vi "WPI_Camera FPS Met.vi"(5 "robot fps":i32 min=0 step=1, 9 "dashboard fps":i32 min=0 step=1) -> (6 "robot fps met?":bool, 10 "dashboard fps met?":bool)   [LabVIEW 2017]
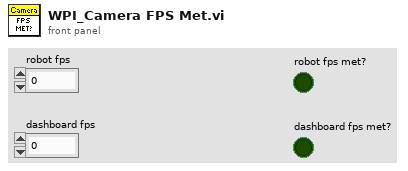
[diagram p1: front panel]
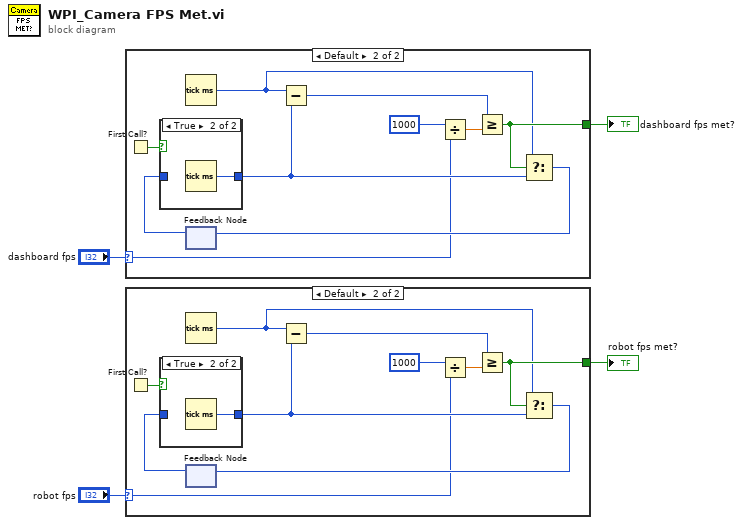
[diagram p0: block diagram]
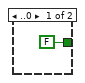
[diagram p2: hidden frame]
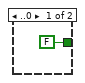
[diagram p4: hidden frame]
diagram:
  n1 = case shown="Default" "dashboard fps" {
    selector: "dashboard fps" -> [_ w6]
    tunnel: [FALSE w10] -> w4
    frame ..0 {
    }
    frame Default {
      n2 = First Call?() -> (First Call?: T/F=w15:bool)
      n3 = Tick Count (ms)() -> (millisecond timer value=w9:u32)
      n4 = feedback #1() -> (w14:u32)  [unwired: 1 in]
      n5 = case shown="True" w15 {
        tunnel: [w16 w17] -> w7
        tunnel: w14 -> [w16 _]
        frame False {
        }
        frame True {
          n6 = Tick Count (ms)() -> (millisecond timer value=w17:u32)
        }
      }
      n7 = Subtract(x=w9, y=w7) -> (x-y=w11:u32)
      n8 = Divide(x=1000 ("robot fps"), y=w6) -> (x/y=w12:dbl)
      n9 = Greater Or Equal?(x=w11, y=w12) -> (x >= y?=w10:bool)
      n10 = Select(t=w9, s=w10, f=w7) -> (s? t:f=w8:u32)
      n11 = feedback-in #1(w8) -> ()
    }
  }
  "dashboard fps met?" <- w4
  n12 = case shown="Default" "robot fps" {
    selector: "robot fps" -> [_ w19]
    tunnel: [FALSE w23] -> w1
    frame ..0 {
    }
    frame Default {
      n13 = First Call?() -> (First Call?: T/F=w28:bool)
      n14 = Tick Count (ms)() -> (millisecond timer value=w22:u32)
      n15 = feedback #2() -> (w27:u32)  [unwired: 1 in]
      n16 = case shown="True" w28 {
        tunnel: [w29 w30] -> w20
        tunnel: w27 -> [w29 _]
        frame False {
        }
        frame True {
          n17 = Tick Count (ms)() -> (millisecond timer value=w30:u32)
        }
      }
      n18 = Subtract(x=w22, y=w20) -> (x-y=w24:u32)
      n19 = Divide(x=1000 ("robot fps"), y=w19) -> (x/y=w25:dbl)
      n20 = Greater Or Equal?(x=w24, y=w25) -> (x >= y?=w23:bool)
      n21 = Select(t=w22, s=w23, f=w20) -> (s? t:f=w21:u32)
      n22 = feedback-in #2(w21) -> ()
    }
  }
  "robot fps met?" <- w1
